vi "main prototype.vi"() -> ()   [LabVIEW 2020]
doc: "Use this template to build a producer/consumer design pattern with events to produce queue items. Use this design pattern instead of the User Interface Event Handler pattern for user interfaces when you want to execute code asynchronously in response to an event without slowing the user interface responsiveness."
panel:
  out "Iterations":i32 caption="Numeric"
  out "Energy":dbl
  out "Velocity":dbl
  out "?":bool
  in  "Save image":bool
  in  "Save data":bool
  out "?":dbl[](graph)
  in  "Reset":bool
  in  "Start":bool
  in  "Stop":bool
  # "Control Panel"
  # "Velocity plot"
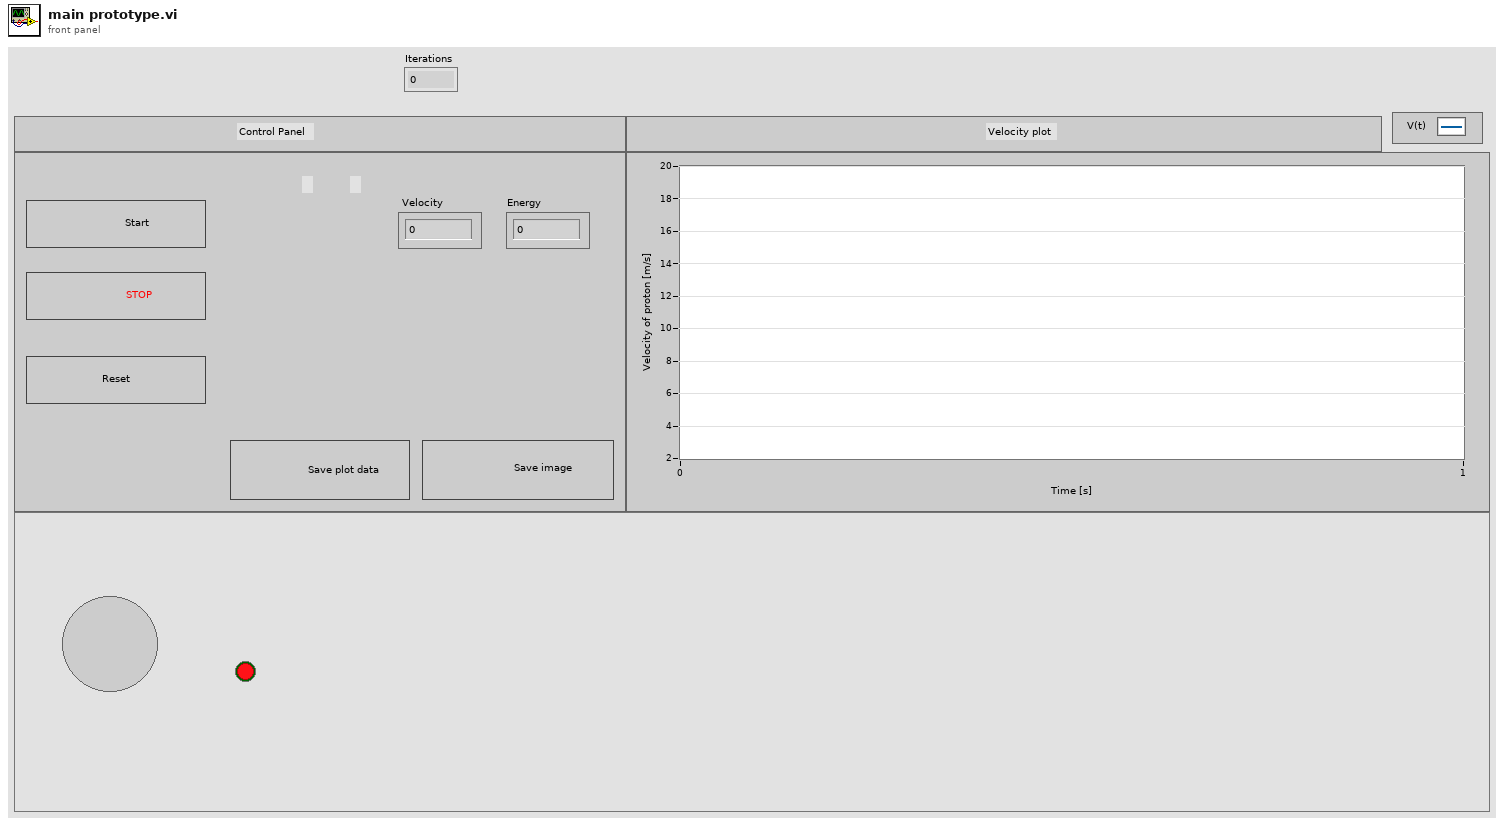
[diagram p1: front panel]
types:
  T1 = enum16{"Default", "Start", "Stop", "Reset", "Save data", "Save image"}
  T2 = cluster{enum16{"Default", "Start", "Stop", "Reset", "Save data", "Save image"}, bool}
  T3 = cluster{enum16{"Default", "Start", "Stop", "Reset", "Save data", "Save image"}, "Stop":bool}
  T4 = cluster{enum16{"Default", "Start", "Stop", "Reset", "Save data", "Save image"}, "Start":bool}
  T5 = cluster{enum16{"Default", "Start", "Stop", "Reset", "Save data", "Save image"}, "Reset":bool}
  T6 = cluster{enum16{"Default", "Start", "Stop", "Reset", "Save data", "Save image"}, "Save data":bool}
  T7 = cluster{enum16{"Default", "Start", "Stop", "Reset", "Save data", "Save image"}, "Save image":bool}
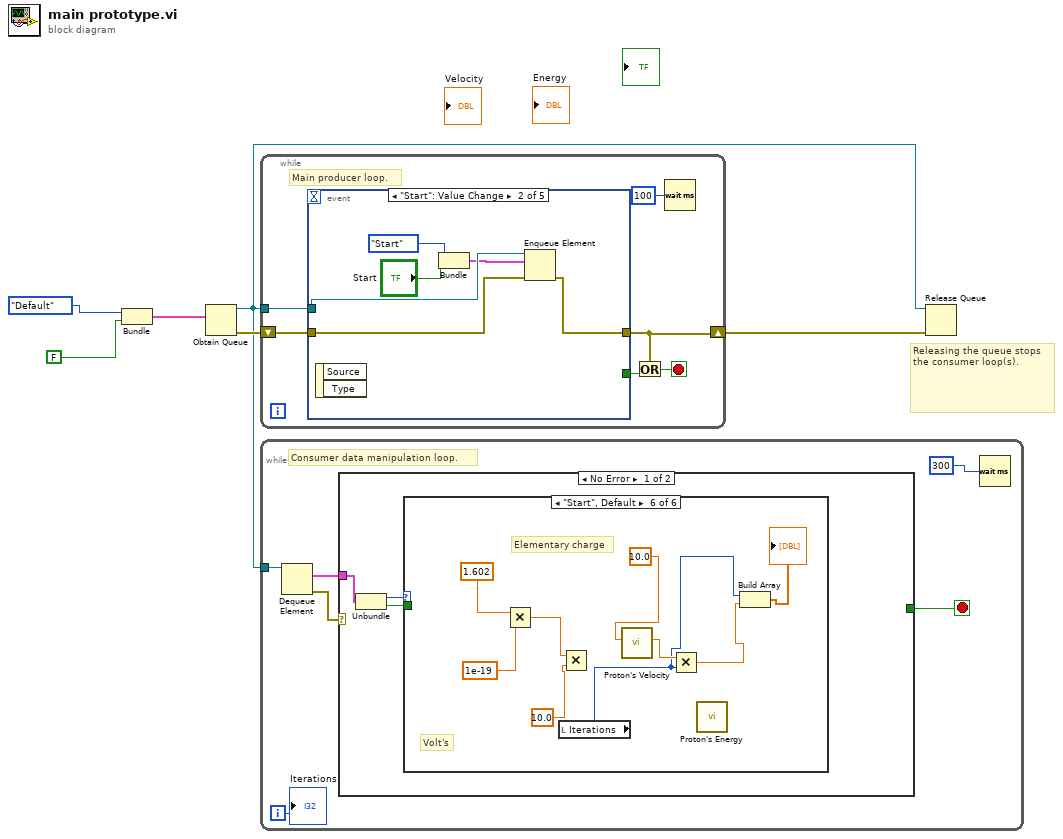
[diagram p0: block diagram]
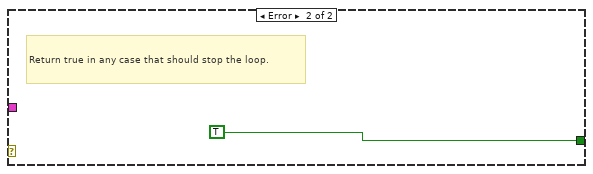
[diagram p7: hidden frame]
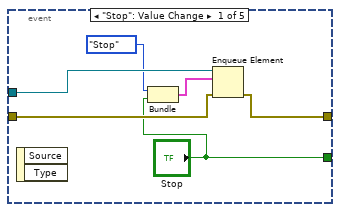
[diagram p8: hidden frame]
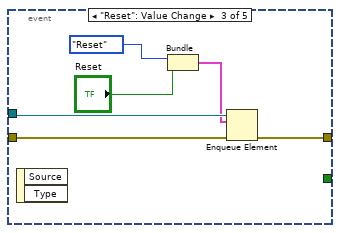
[diagram p9: hidden frame]
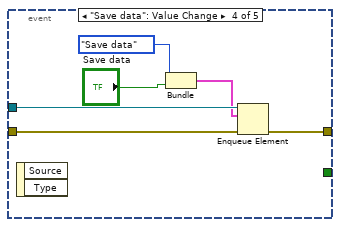
[diagram p10: hidden frame]
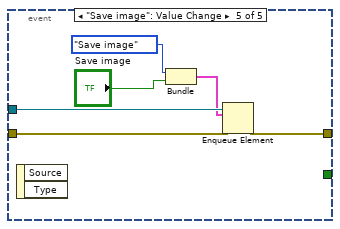
[diagram p11: hidden frame]
diagram:
  # "Releasing the queue stops the consumer loop(s)."
  n1 = Bundle(T1."Default", FALSE) -> (w2:T2)  [unwired: 1 in]
  n2 = Obtain Queue(element data type=w2) -> (queue out=w4:refnum<queue>, error out=w6:errorcluster)  [unwired: 4 in, 1 out]
  n3 = while {
    shift-right: [w8] -> w5
    shift-left: w6 -> [w11]
    tunnel: w4 -> [w12]
    stop <- w9 stop-if-true
    # "Main producer loop."
    n4 = event shown="[1] \"Start\": Value Change" {
      selector: _ -> [_ _ _ _ _]
      dyn-events: _ -> [_ _ _ _ _]
      timeout: _ -> [_ _ _ _ _]
      tunnel: w12 -> [w18 w24 w30 w36 w42]
      tunnel: w11 -> [w17 w20 w26 w31 w38]
      tunnel: [w16 w19 w25 w32 w37] -> w8
      tunnel: ["Stop" _ _ _ _] -> w10
      event "Stop": Value Change {
        n5 = event-data() -> ()  [unwired: 1 in, 2 out]
        n6 = Bundle(T1."Stop", "Stop"="Stop") -> (w15:T3)  [unwired: 1 in]
        n7 = Enqueue Element(queue=w18, element=w15, error in (no error)=w17) -> (error out=w16:errorcluster)  [unwired: 1 in, 2 out]
      }
      event "Start": Value Change {
        n8 = event-data() -> ()  [unwired: 1 in, 2 out]
        n9 = Bundle(T1."Start", "Start"="Start") -> (w22:T4)  [unwired: 1 in]
        n10 = Enqueue Element(queue=w24, element=w22, error in (no error)=w20) -> (error out=w19:errorcluster)  [unwired: 1 in, 2 out]
      }
      event "Reset": Value Change {
        n11 = event-data() -> ()  [unwired: 1 in, 2 out]
        n12 = Bundle(T1."Reset", "Reset"="Reset") -> (w28:T5)  [unwired: 1 in]
        n13 = Enqueue Element(queue=w30, element=w28, error in (no error)=w26) -> (error out=w25:errorcluster)  [unwired: 1 in, 2 out]
      }
      event "Save data": Value Change {
        n14 = event-data() -> ()  [unwired: 1 in, 2 out]
        n15 = Bundle(T1."Save data", "Save data"="Save data") -> (w35:T6)  [unwired: 1 in]
        n16 = Enqueue Element(queue=w36, element=w35, error in (no error)=w31) -> (error out=w32:errorcluster)  [unwired: 1 in, 2 out]
      }
      event "Save image": Value Change {
        n17 = event-data() -> ()  [unwired: 1 in, 2 out]
        n18 = Bundle(T1."Save image", "Save image"="Save image") -> (w39:T7)  [unwired: 1 in]
        n19 = Enqueue Element(queue=w42, element=w39, error in (no error)=w38) -> (error out=w37:errorcluster)  [unwired: 1 in, 2 out]
      }
    }
    n20 = Or(x=w8, y=w10) -> (x .or. y?=w9:bool)
    n21 = Wait (ms)(milliseconds to wait=u32 100) -> ()  [unwired: 1 out]
  }
  n22 = while {
    tunnel: w4 -> [w48]
    i -> [w43]
    stop <- w45 stop-if-true
    # "Consumer data manipulation loop."
    n23 = Dequeue Element(queue=w48) -> (element=w46:T2, error out=w47:errorcluster)  [unwired: 2 in, 2 out]
    n24 = case shown="No Error" w47 {
      tunnel: w46 -> [w51 _]
      tunnel: [_ TRUE] -> w45
      frame No Error {
        n25 = Unbundle(w51) -> (w49:T1, w50:bool)
        n26 = case shown="\"Start\", Default" w49 {
          tunnel: w50 -> [_ _ _ _ _ _]
          frame "Stop" {
          }
          frame "Reset" {
          }
          frame "Save data" {
          }
          frame "Save image" {
          }
          frame "Default" {
          }
          frame "Start", Default {
            # "Volt's"
            # "Elementary charge"
            n27 = Multiply(x=1.602, y=1e-19) -> (x*y=w58:dbl)
            n28 = local read "Iterations"() -> (w54:i32)
            n29 = Multiply(x=w58, y=10.0) -> ()  [unwired: 1 out]
            n30 = call "Proton's Velocity.vi"("Starting Velocity"=10.0) -> ("Velocity"=w55:dbl)  [unwired: 10 in]
            n31 = Multiply(x=w55, y=w54) -> (x*y=w53:dbl)
            n32 = call "Proton's Energy.vi"() -> ()  [unwired: 11 in, 1 out]
            n33 = Build Array(w54, w53) -> (→"?":dbl[])
          }
        }
      }
      frame Error {
        # "Return true in any case that should stop the loop."
      }
    }
    n34 = Wait (ms)(milliseconds to wait=u32 300) -> ()  [unwired: 1 out]
    "Iterations" <- w43
  }
  n35 = Release Queue(queue=w4, error in (no error)=w5) -> ()  [unwired: 1 in, 3 out]
